vi "BRig_dataMTrig_init.vi"() -> (2 "output_dataMTrig":u16[](array[numeric]))   [LabVIEW 2014]
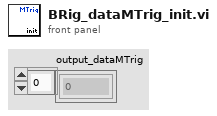
[diagram p1: front panel]
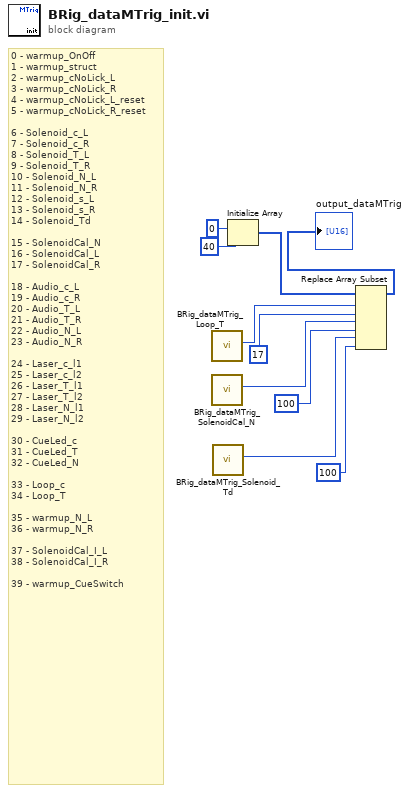
[diagram p0: block diagram]
diagram:
  # "0 - warmup_OnOff\n1 - warmup_struct\n2 - warmup_cNoLick_L\n3 - warmup_cNoLick_R\n4 - warmup_cNoLick_L_reset\n5 - warmup_cNoLick_R_reset\n\n6 - Solenoid_c_L\n7 - Solenoid_c_R\n8 - Solenoid_T_L\n9 - Solenoid_T_R\n10 - Solenoid_N_L\n11 - Solenoid_N_R\n12 - Solenoid_s_L\n13 - Solenoid_s_R\n14 - Solenoid_Td\n\n15 - SolenoidCal_N\n16 - SolenoidCal_L\n17 - SolenoidCal_R\n\n18 - Audio_c_L\n19 - Audio_c_R\n20 - Audio_T_L\n21 - Audio_T_R\n22 - Audio_N_L\n23 - Audio_N_R\n\n24 - Laser_c_l1\n25 - Laser_c_l2\n26 - Laser_T_l1\n27 - Laser_T_l2\n28 - Laser_N_l1\n29 - Laser_N_l2\n\n30 - CueLed_c\n31 - CueLed_T\n32 - CueLed_N\n\n33 - Loop_c\n34 - Loop_T\n\n35 - warmup_N_L\n36 - warmup_N_R\n\n37 - SolenoidCal_I_L\n38 - SolenoidCal_I_R\n\n39 - warmup_CueSwitch"
  n1 = call "BRig_dataMTrig_Loop_T.vi"() -> ("output_Loop_T"=w6:i32)  [unwired: 11 in]
  n2 = call "BRig_dataMTrig_SolenoidCal_N.vi"() -> ("output_SolenoidCal_N"=w4:i32)  [unwired: 11 in]
  n3 = call "BRig_dataMTrig_Solenoid_Td.vi"() -> ("output_Solenoid_Td"=w2:i32)  [unwired: 11 in]
  n4 = Initialize Array(u16 0 ("element"), 40 ("dimension size")) -> (w8:u16[])
  n5 = Replace Array Subset(array=w8, new element #1=u16 17 ("new element/subarray"), index #1=w6, new element #2=u16 100 ("new element/subarray"), index #2=w4, new element #3=u16 100 ("new element/subarray"), index #3=w2) -> (→"output_dataMTrig":u16[])
